vi "Record Data.vi"(3 "Voltage":dynamicdata(graph), 9 "Continuous Rec Data CH0":bool, 10 "Record single value":bool, 11 "Select path and filename":path) -> ()   [LabVIEW 2012]
uses:
  <vilib>/Waveform/WDTFileIO.llb/ Write Waveforms to File (1D).vi
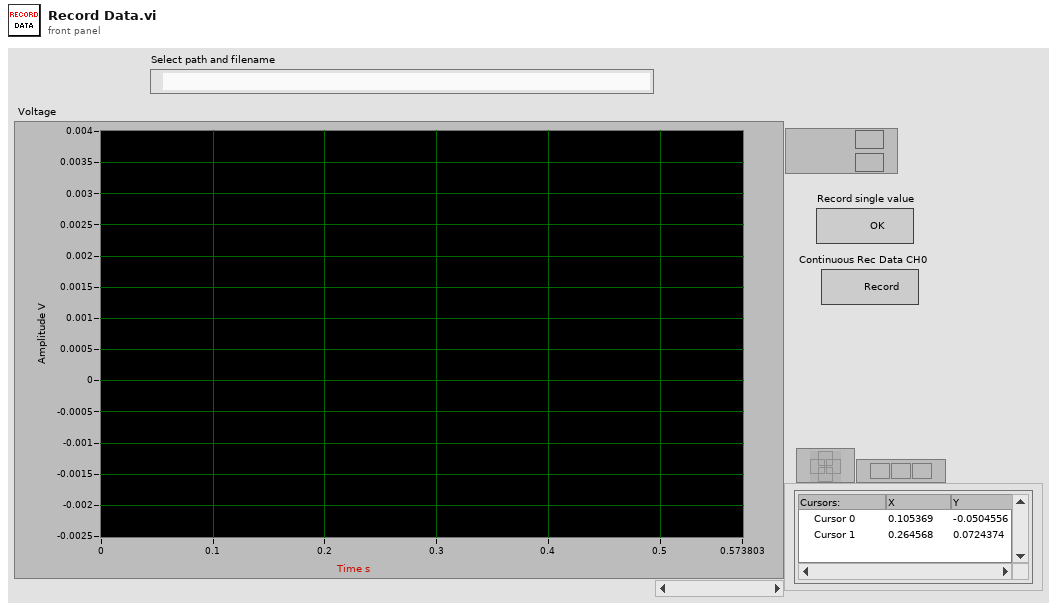
[diagram p1: front panel]
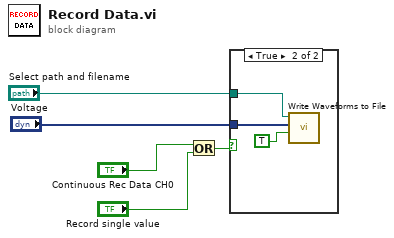
[diagram p0: block diagram]
diagram:
  n1 = Or(x="Continuous Rec Data CH0", y="Record single value") -> (x .or. y?=w3:bool)
  n2 = case shown="True" w3 {
    tunnel: "Voltage" -> [_ w8]
    tunnel: "Select path and filename" -> [_ w6]
    frame False {
    }
    frame True {
      n3 = call-poly <vilib>:"Write Waveforms to File.vi"("append to file? (new file:F)"=TRUE, "waveform array"=w8, "file path (dialog if empty)"=w6) -> ()  [unwired: 7 in, 2 out]
    }
  }
